vi "writeToXML.vi"(8 "error in (no error)":errorcluster, 10 "Class Label":string="RotatorPositions", 11 "RotatorPositions in":refnum<class "RotatorPositions.lvclass">) -> (0 "error out":errorcluster, 2 "XML out":string="<RotatorPosition>\n  <rotPA>0</rotPA>\n</RotatorPosition>", 3 "RotatorPositions out":refnum<class "RotatorPositions.lvclass">)   [LabVIEW 2014, in "TCSDataDefinitions.lvlib" / "TCSPublicStatus.lvlib" / "PointingPositions.lvlib" / "RotatorPositions.lvclass"]
uses:
  RotatorPositions.lvclass
  <userlib>/Common/UnitsAndXML/FlattenItemWithUnitToXML/FlattenPlaneAngleToXML/PlaneAngleUnit.ctl
  RotatorPositions.lvclass/RotatorPositions.ctl
  <userlib>/Common/UnitsAndXML/UnitsAndXML.lvlib
  <userlib>/Common/XML/XMLGenerator/XMLGenerator.lvclass
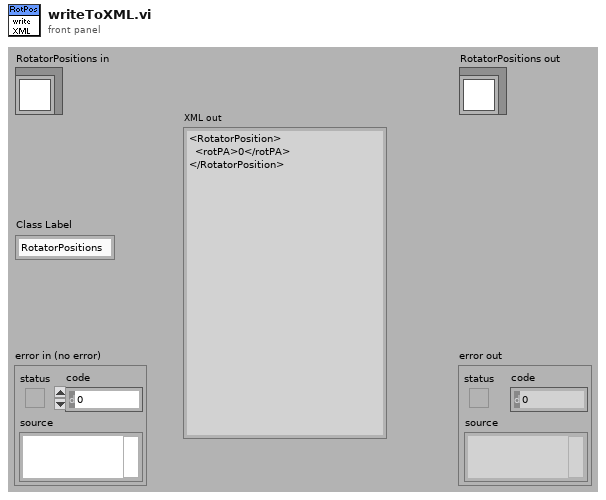
[diagram p1: front panel]
types:
  T1 = typedef "UnitsAndXML.lvlib/PlaneAngleUnit.ctl" = enum16{"rad", "deg", "'", "\""}
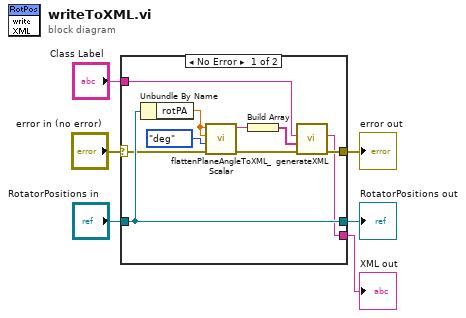
[diagram p0: block diagram]
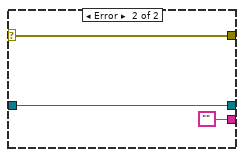
[diagram p2: hidden frame]
diagram:
  n1 = case shown="No Error" "error in (no error)" {
    selector: "error in (no error)" -> [w13 w19]
    tunnel: [w10 w19] -> w5
    tunnel: [w16 w18] -> w1
    tunnel: "RotatorPositions in" -> [w16 w18]
    tunnel: "Class Label" -> [w7 _]
    tunnel: [w9 ""] -> w3
    frame No Error {
      n2 = Unbundle By Name(w16) -> ("rotPA"=w15:dbl[unit])
      n3 = call <userlib>:"flattenPlaneAngleToXML_Scalar.vi"("error in (no error)"=w13, "planeAngleUnitInXML"=PlaneAngleUnit."deg", "planeAngleAgain"=w15, "planeAngle"=w15) -> ("error out"=w11:errorcluster, "xmlString"=w12:string)  [unwired: 6 in]
      n4 = Build Array(w12) -> (w8:string[])
      n5 = call <userlib>:"generateXML.vi"("error in"=w11, "childrenXML"=w8, "elementName"=w7) -> ("error out"=w10:errorcluster, "XML out"=w9:string)  [unwired: 6 in, 1 out]
    }
    frame Error {
    }
  }
  "error out" <- w5
  "XML out" <- w3
  "RotatorPositions out" <- w1
